vi "StepperData.vi"() -> ()   [LabVIEW 2014]
panel:
  out "Flipping i":i32
  out "Loop i":i32
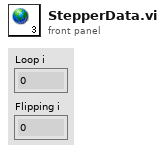
[diagram p1: front panel]
diagram:
